vi "2024_day09_Task02.vi"() -> ()   [LabVIEW 2023]
uses:
  <userlib>/_OpenG.lib/array/array.llb/Search 1D Array (I32)__ogtk.vi
  <userlib>/_OpenG.lib/array/array.llb/Delete Elements from 1D Array (I32)__ogtk.vi
  <userlib>/_OpenG.lib/string/string.llb/openg_string.lvlib
  <userlib>/_OpenG.lib/array/array.llb/openg_array.lvlib
panel:
  out "FILES":i32[](array[numeric])
  out "SPACES":i32[](array[numeric])
  out "Array 3":i32[](array[numeric])
  out "Array 2":i32[](array[numeric])
  out "Array":i32[](array[numeric])
  out "Result - Task 2":i64
  in  "Switch":bool caption="Ex. Data  vs.  User Data"
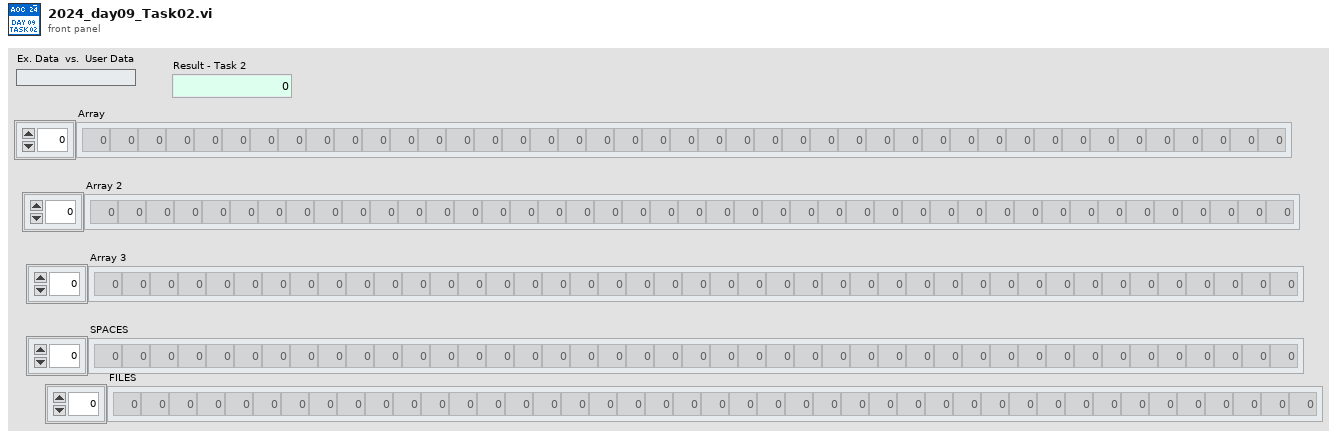
[diagram p1: front panel]
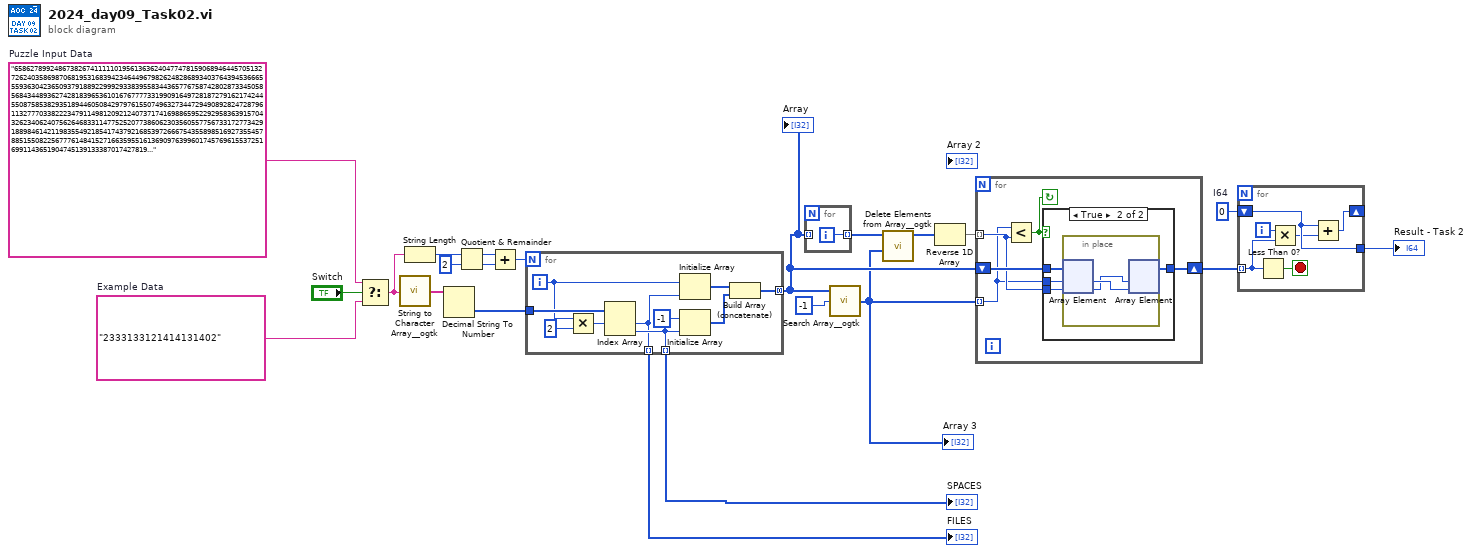
[diagram p0: block diagram]
diagram:
  w6 = i64 0  # I64
  w20 = "658627899248673826741111101956136362404774781590689464457051327262403586987068195316839423464496798262482868934037643945366655593630423650937918892299929338395583443657767587428028733450585684344893627428183965361016767777331990916497281872791621742445508758538293518944605084297976155074963273447294908928247287961132777033822234791149812092124073717416988659522929583639157043262340624075626468331147752520773860623035605577567331727734291889846142119835549218541743792168539726667543558985169273554578851550822567776148415271663595516136909763996017457696155372516991143651904745139133387017427819..."  # Puzzle Input Data
  w21 = "2333133121414131402"  # Example Data
  n1 = Select(t=w20, s="Switch", f=w21) -> (s? t:f=w18:string)
  n2 = call <userlib>:"String to Character Array__ogtk.vi"("Input String"=w18) -> ("Character Array"=w19:string[])
  n3 = String Length(string=w18) -> (length=w17:i32)
  n4 = Decimal String To Number(string=w19) -> (number=w14:i32[])  [unwired: 2 in, 1 out]
  n5 = Quotient & Remainder(x=w17, y=2) -> (x-y*floor(x/y)=w12:i32, floor(x/y)=w15:i32)
  n6 = Add(x=w12, y=w15) -> (x+y=w13:i32)
  n7 = for {
    N: w13 -> [_]
    tunnel: [w29] -> w9 mode=concatenating
    tunnel: w14 -> [w28]
    tunnel: [w24] -> w2 mode=indexing
    tunnel: [w23] -> w1 mode=indexing
    i -> [w27]
    n8 = Multiply(x=w27, y=2) -> (x*y=w26:i32)
    n9 = Index Array(array=w28, index #1=w26) -> (element #1=w23:i32, element #2=w24:i32)  [unwired: 1 in]
    n10 = Initialize Array(w27, w23) -> (w32:i32[])
    n11 = Initialize Array(-1 ("element"), w24) -> (w31:i32[])
    n12 = Build Array (concatenate)(w32, w31) -> (w29:i32[])
  }
  "Array" <- w9
  "SPACES" <- w2
  "FILES" <- w1
  n13 = for {
    tunnel: [w33] -> w8 mode=indexing
    tunnel: w9 -> [_] mode=indexing
    i -> [w33]
  }
  n14 = call-poly <userlib>:"Search Array__ogtk.vi"("Array"=w9, "Element Data"=-1) -> ("Indices of Elements"=w3:i32[])  [unwired: 7 in]
  "Array 3" <- w3
  n15 = call-poly <userlib>:"Delete Elements from Array__ogtk.vi"("indices"=w3, "array"=w8) -> ("array w/ subset deleted"=w4:i32[])  [unwired: 8 in, 1 out]
  n16 = Reverse 1D Array(array=w4) -> (reversed array=w7:i32[])
  n17 = for {
    tunnel: w3 -> [w35] mode=indexing
    shift-right: [w37] -> w10
    shift-left: w9 -> [w38]
    tunnel: w7 -> [w36] mode=indexing
    stop <- w34 continue-if-true
    n18 = Less?(x=w35, y=w36) -> (x < y?=w34:bool)
    n19 = case shown="True" w34 {
      tunnel: w38 -> [w39 w43]
      tunnel: [w39 w42] -> w37
      tunnel: w36 -> [_ w41]
      tunnel: w35 -> [_ w40]
      frame False {
      }
      frame True {
        n20 = in-place {
          n21 = in-place-array #1(w43, w40, w41) -> (w45:i32, w44:i32)
          n22 = in-place-array #1(w44, w45) -> (w42:i32[])  [unwired: 2 out]
        }
      }
    }
  }
  n23 = for {
    tunnel: w10 -> [w50] mode=indexing
    shift-right: [w46] -> _
    shift-left: w6 -> [w48]
    tunnel: [w48] -> w5
    i -> [w49]
    stop <- w51 stop-if-true
    n24 = Less Than 0?(x=w50) -> (x < 0?=w51:bool)
    n25 = Multiply(x=w49, y=w50) -> (x*y=w47:i32)
    n26 = Add(x=w48, y=w47) -> (x+y=w46:i64)
  }
  "Result - Task 2" <- w5
